vi "type_casting.vi"() -> ()   [LabVIEW 2013, in "TCP_IP.lvclass"]
uses:
  TCP_IP.lvclass
panel:
  out "output array":u16[][][](array[numeric])
  out "*(type *) &x 2":u16[](array[numeric])
  out "*(type *) &x":string
  in  "Array of U16 from last measurement (shots,x,y)":u16[][][](array[numeric])
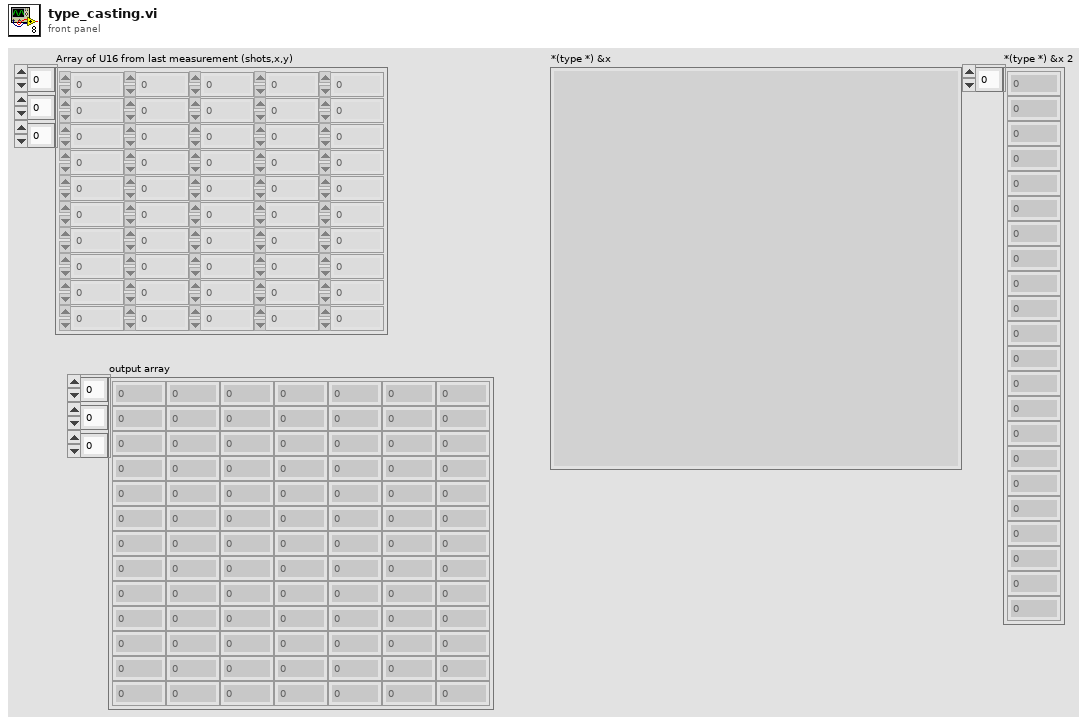
[diagram p1: front panel]
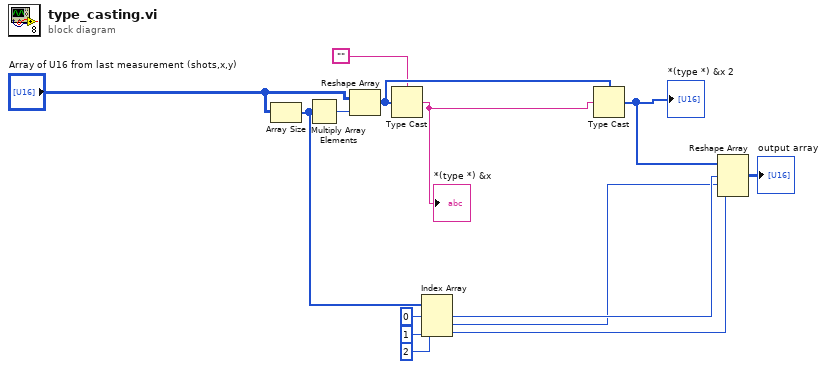
[diagram p0: block diagram]
diagram:
  n1 = Array Size(array="Array of U16 from last measurement (shots,x,y)") -> (size(s)=w8:i32[])
  n2 = Multiply Array Elements(1:w8) -> (0:w14:i32)
  n3 = Reshape Array("Array of U16 from last measurement (shots,x,y)", w14) -> (w11:u16[])
  n4 = Type Cast(type="", x=w11) -> (*(type *) &x=w12:string)
  "*(type *) &x" <- w12
  n5 = Index Array(array=w8, index #1=0 ("index"), index #2=1 ("index"), index #3=2 ("index")) -> (element #1=w6:i32, element #2=w3:i32, element #3=w2:i32)
  n6 = Type Cast(type=w11, x=w12) -> (*(type *) &x=w9:u16[])
  "*(type *) &x 2" <- w9
  n7 = Reshape Array(w9, w6, w3, w2) -> (→"output array":u16[][][])
